vi "Classfy.vi"() -> (0 "Classfy 1":T1[](array[typedef])=[{"Item"="¤C¤H¨î¾ñÆV²y", "Count"=2, "Athletics"=["¨k¤l¤C¤H¨î¾ñÆV²y", "¤k¤l¤C¤H¨î¾ñÆV²y"]}, {"Item"="¤p½ü¨®", "Count"=2, "Athletics"=["¨k¤l­Ó¤H¤p½ü¨®", "¤k¤l­Ó¤H¤p½ü¨®"]}, {"Item"="¤½¸ô¦Û¥Ñ¨®", "Count"=4, "Athletics"=["¤k¤l­p®ÉÁÉ¤½¸ô¦Û¥Ñ¨®", "¨k¤l­p®ÉÁÉ¤½¸ô¦Û¥Ñ¨®", "¨k¤l¤½¸ôÁÉ¤½¸ô¦Û¥Ñ¨®", "¤k¤l¤½¸ôÁÉ¤½¸ô¦Û¥Ñ¨®"]}, {"Item"="¤â²y", "Count"=2, "Athletics"=["¨k¤l¤â²y", "¤k¤l¤â²y"]}, {"Item"="¤ô¤WªÝÁ¢", "Count"=2, "Athletics"=["¤k¤lÂù¤H¤ô¤WªÝÁ¢", "¤k¤l¹ÎÅé¤ô¤WªÝÁ¢"]}, {"Item"="¤ô²y", "Count"=2, "Athletics"=["¨k¤l¤ô²y", "¤k¤l¤ô²y"]}, {"Item"="¥Ð®|", "Count"=47, "Athletics"=["¨k¤l100¤½¤Ø", "¨k¤l200¤½¤Ø", "¨k¤l400¤½¤Ø", "¨k¤l800¤½¤Ø", "¨k¤l1500¤½¤Ø", "¨k¤l5000¤½¤Ø", "¨k¤l10,000¤½¤Ø", "¨k¤l110¤½¤Ø¸óÄæ", "¨k¤l400¤½¤Ø¸óÄæ", "¨k¤l3000¤½¤Ø»ÙÃª", "¨k¤l4¡Ñ100¤½¤Ø±µ¤O", "¨k¤l4¡Ñ400¤½¤Ø±µ¤O", "¨k¤l°¨©ÔªQ", "¨k¤l20¤½¨½Äv¨«", "¨k¤l50¤½¨½Äv¨«", "¨k¤l¸õ°ª", "¨k¤l¼µ¬ñ¸õ°ª", "¨k¤l¸õ»·", "¨k¤l¤T¯Å¸õ»·", "¨k¤l¹]²y", "¨k¤lÅK»æ", "¨k¤lÃì²y", "¨k¤l¼Ðºj", "¨k¤l¤Q¶µ¥þ¯à", "¤k¤l100¤½¤Ø", "¤k¤l200¤½¤Ø", "¤k¤l400¤½¤Ø", "¤k¤l800¤½¤Ø", "¤k¤l1500¤½¤Ø", "¤k¤l5000¤½¤Ø", "¤k¤l10,000¤½¤Ø", "¤k¤l100¤½¤Ø¸óÄæ", "¤k¤l400¤½¤Ø¸óÄæ", "¤k¤l3000¤½¤Ø»ÙÃª", "¤k¤l4¡Ñ100¤½¤Ø±µ¤O", "¤k¤l4¡Ñ400¤½¤Ø±µ¤O", "¤k¤l°¨©ÔªQ", "¤k¤l20¤½¨½Äv¨«", "¤k¤l¸õ°ª", "¤k¤l¼µ¬ñ¸õ°ª", "¤k¤l¸õ»·", "¤k¤l¤T¯Å¸õ»·", "¤k¤l¹]²y", "¤k¤lÅK»æ", "¤k¤lÃì²y", "¤k¤l¼Ðºj", "¤k¤l¤C¶µ¥þ¯à"]}, {"Item"="¦E²î", "Count"=14, "Athletics"=["¨k¤l³æ¤HÂù¼Õ", "¨k¤lÂù¤H³æ¼Õ", "¨k¤lÂù¤HÂù¼Õ", "¨k¤l¥|¤H³æ¼Õ", "¨k¤l¥|¤HÂù¼Õ", "¨k¤l¤K¤H³æ¼Õ", "¨k¤l»´¶q¯ÅÂù¤HÂù¼Õ", "¨k¤l»´¶q¯Å¥|¤H³æ¼Õ", "¤k¤l³æ¤HÂù¼Õ", "¤k¤lÂù¤H³æ¼Õ", "¤k¤lÂù¤HÂù¼Õ", "¤k¤l¥|¤HÂù¼Õ", "¤k¤l¤K¤H³æ¼Õ", "¤k¤l»´¶q¯ÅÂù¤HÂù¼Õ"]}, {"Item"="¦|²î", "Count"=10, "Athletics"=["¤k¤lRS¡GX«¬¡]­·®öªO¡^", "¤k¤l¹p®g¿ç®g«¬¡]³æ¤H¸¥¡^", "¤k¤l470«¬¡]Âù¤H¸¥¡^", "¤k¤l49¤H«¬FX¡]§Ö¸¥¡^", "¨k¤lRS¡GX«¬¡]­·®öªO¡^", "¨k¤l¹p®g«¬¡]³æ¤H¸¥¡^", "¨k¤lªâÄõ¤H«¬¡]³æ¤H¸¥¡^", "¨k¤l470«¬¡]Âù¤H¸¥¡^", "¨k¤l49¤H«¬¡]§Ö¸¥¡^", "²V¦XNacra17«¬¡]¦hÅé²î¡^"]}, {"Item"="¦±´Ò²y", "Count"=2, "Athletics"=["¨k¤l¦±´Ò²y", "¤k¤l¦±´Ò²y"]}, {"Item"="¦Ð²y", "Count"=5, "Athletics"=["²V¦XÂù¥´¦Ð²y", "¨k¤lÂù¥´¦Ð²y", "¤k¤lÂù¥´¦Ð²y", "¨k¤l³æ¥´¦Ð²y", "¤k¤l³æ¥´¦Ð²y"]}, {"Item"="¨FÅy±Æ²y", "Count"=2, "Athletics"=["¨k¤l¨FÅy±Æ²y", "¤k¤l¨FÅy±Æ²y"]}, {"Item"="¨¤¤O", "Count"=18, "Athletics"=["¨k¤l§ÆÃ¹¦¡59¤½¤ç¯Å", "¨k¤l§ÆÃ¹¦¡66¤½¤ç¯Å", "¨k¤l§ÆÃ¹¦¡75¤½¤ç¯Å", "¨k¤l§ÆÃ¹¦¡85¤½¤ç¯Å", "¨k¤l§ÆÃ¹¦¡98¤½¤ç¯Å", "¨k¤l§ÆÃ¹¦¡130¤½¤ç¯Å", "¨k¤l¦Û¥Ñ¦¡57¤½¤ç¯Å", "¨k¤l¦Û¥Ñ¦¡65¤½¤ç¯Å", "¨k¤l¦Û¥Ñ¦¡74¤½¤ç¯Å", "¨k¤l¦Û¥Ñ¦¡86¤½¤ç¯Å", "¨k¤l¦Û¥Ñ¦¡97¤½¤ç¯Å", "¨k¤l¦Û¥Ñ¦¡125¤½¤ç¯Å", "¤k¤l¦Û¥Ñ¦¡48¤½¤ç¯Å", "¤k¤l¦Û¥Ñ¦¡53¤½¤ç¯Å", "¤k¤l¦Û¥Ñ¦¡58¤½¤ç¯Å", "¤k¤l¦Û¥Ñ¦¡63¤½¤ç¯Å", "¤k¤l¦Û¥Ñ¦¡69¤½¤ç¯Å", "¤k¤l¦Û¥Ñ¦¡75¤½¤ç¯Å"]}, {"Item"="¨¬²y", "Count"=2, "Athletics"=["¨k¤l¨¬²y", "¤k¤l¨¬²y"]}, {"Item"="¬X¹D", "Count"=14, "Athletics"=["¨k¤l60¤½¤ç¯Å¬X¹D", "¨k¤l66¤½¤ç¯Å¬X¹D", "¨k¤l73¤½¤ç¯Å¬X¹D", "¨k¤l81¤½¤ç¯Å¬X¹D", "¨k¤l90¤½¤ç¯Å¬X¹D", "¨k¤l100¤½¤ç¯Å¬X¹D", "¨k¤l100¤½¤ç¥H¤W¯Å¬X¹D", "¤k¤l48¤½¤ç¯Å¬X¹D", "¤k¤l52¤½¤ç¯Å¬X¹D", "¤k¤l57¤½¤ç¯Å¬X¹D", "¤k¤l63¤½¤ç¯Å¬X¹D", "¤k¤l70¤½¤ç¯Å¬X¹D", "¤k¤l78¤½¤ç¯Å¬X¹D", "¤k¤l78¤½¤ç¥H¤W¯Å¬X¹D"]}, {"Item"="®g½b", "Count"=4, "Athletics"=["¨k¤l­Ó¤H®g½b", "¤k¤l­Ó¤H®g½b", "¨k¤l¹ÎÅé®g½b", "¤k¤l¹ÎÅé®g½b"]}, {"Item"="®gÀ»", "Count"=15, "Athletics"=["¨k¤l10¤½¤ØªÅ®ð¤âºj", "¨k¤l10¤½¤ØªÅ®ð¨Bºj", "¨k¤l25¤½¤Ø§Ö®g¤âºj", "¨k¤l50¤½¤Ø¤âºj", "¨k¤l50¤½¤Ø¨Bºjª×«º", "¨k¤l50¤½¤Ø¨Bºj¤T«º", "¨k¤l©w¦V­¸¹v", "¨k¤l¤£©w¦V­¸¹v", "¨k¤lÂù¤£©w¦V­¸¹v", "¤k¤l10¤½¤ØªÅ®ð¤âºj", "¤k¤l10¤½¤ØªÅ®ð¨Bºj", "¤k¤l25¤½¤Ø¤âºj", "¤k¤l50¤½¤Ø¨Bºj¤T«º", "¤k¤l©w¦V­¸¹v", "¤k¤l¤£©w¦V­¸¹v"]}, {"Item"="®±À»", "Count"=13, "Athletics"=["¨k¤l»´ÃÇ¶q49¤½¤ç¯Å", "¨k¤lÃÇ¶q52¤½¤ç¯Å", "¨k¤lÂú¶q56¤½¤ç¯Å", "¨k¤l»´¶q60¤½¤ç¯Å", "¨k¤l»´¨I¶q64¤½¤ç¯Å", "¨k¤l¨I¶q69¤½¤ç¯Å", "¨k¤l¤¤¶q75¤½¤ç¯Å", "¨k¤l»´­«¶q81¤½¤ç¯Å", "¨k¤l­«¶q91¤½¤ç¯Å", "¨k¤l¶W­«¶q91¤½¤ç¥H¤W¯Å", "¤k¤lÃÇ¶q51¤½¤ç¯Å", "¤k¤l»´¶q60¤½¤ç¯Å", "¤k¤l¤¤¶q75¤½¤ç¯Å"]}, {"Item"="®à²y", "Count"=4, "Athletics"=["¨k¤l³æ¥´®à²y", "¤k¤l³æ¥´®à²y", "¨k¤l¹ÎÅé®à²y", "¤k¤l¹ÎÅé®à²y"]}, {"Item"="°¨³N", "Count"=6, "Athletics"=["¹ÎÅé²±¸Ë»R¨BÁÉ", "­Ó¤H²±¸Ë»R¨BÁÉ", "­Ó¤H¤T¶µÁÉ", "¹ÎÅé¤T¶µÁÉ", "¹ÎÅé³õ¦a»ÙÃªÁÉ", "­Ó¤H³õ¦a»ÙÃªÁÉ"]}, {"Item"="蔼焊ひ", "Count"=2, "Athletics"=["¤k¤l­Ó¤H°ªº¸¤Ò", "¨k¤l­Ó¤H°ªº¸¤Ò"]}, {"Item"="±Æ²y", "Count"=2, "Athletics"=["¤k¤l±Æ²y", "¨k¤l±Æ²y"]}, {"Item"="²{¥N¤­¶µ", "Count"=2, "Athletics"=["¨k¤l­Ó¤H²{¥N¤­¶µ", "¤k¤l­Ó¤H²{¥N¤­¶µ"]}, {"Item"="³õ¦a¦Û¥Ñ¨®", "Count"=10, "Athletics"=["¨k¤l¹ÎÅéª§¥ýÁÉ", "¤k¤l¹ÎÅé°l³vÁÉ", "¨k¤l¹ÎÅé°l³vÁÉ", "¤k¤l¹ÎÅéª§¥ýÁÉ", "¨k¤lª§¥ýÁÉ", "¤k¤l°l³vÁÉ", "¨k¤l°l³vÁÉ", "¤k¤lª§¥ýÁÉ", "¨k¤l¥þ¯à", "¤k¤l¥þ¯à"]}, {"Item"="´åªa", "Count"=34, "Athletics"=["¨k¤l±¶ªa¡G50¤½¤Ø¡B100¤½¤Ø¡B200¤½¤Ø¡B400¤½¤Ø¡B1500¤½¤Ø", "¤k¤l±¶ªa¡G50¤½¤Ø¡B100¤½¤Ø¡B200¤½¤Ø¡B400¤½¤Ø¡B800¤½¤Ø", "¨k¤l¥õ¦¡¡G100¤½¤Ø¡B200¤½¤Ø", "¤k¤l¥õ¦¡¡G100¤½¤Ø¡B200¤½¤Ø", "¨k¤lµì¦¡¡G100¤½¤Ø¡B200¤½¤Ø", "¤k¤lµì¦¡¡G100¤½¤Ø¡B200¤½¤Ø", "¨k¤l½º¦¡¡G100¤½¤Ø¡B200¤½¤Ø", "¤k¤l½º¦¡¡G100¤½¤Ø¡B200¤½¤Ø", "¨k¤l²V¦X¦¡¡G200¤½¤Ø¡B400¤½¤Ø", "¤k¤l²V¦X¦¡¡G200¤½¤Ø¡B400¤½¤Ø", "¨k¤l±¶ªa±µ¤O¡G4¡Ñ100¤½¤Ø¡B4¡Ñ200¤½¤Ø", "¤k¤l±¶ªa±µ¤O¡G4¡Ñ100¤½¤Ø¡B4¡Ñ200¤½¤Ø", "¨k¤l²V¦X¦¡±µ¤O¡G4¡Ñ100¤½¤Ø", "¤k¤l²V¦X¦¡±µ¤O¡G4¡Ñ100¤½¤Ø", "¨k¤l¤½¶}¤ô°ì´åªa¡G10¤½¨½", "¤k¤l¤½¶}¤ô°ì´åªa¡G10¤½¨½"]}, {"Item"="µn¤s¦Û¥Ñ¨®", "Count"=2, "Athletics"=["¨k¤l¶V³¥ÁÉ", "¤k¤l¶V³¥ÁÉ"]}, {"Item"="¶`®±¹D", "Count"=8, "Athletics"=["¨k¤l58¤½¤ç¯Å¶`®±¹D", "¨k¤l68¤½¤ç¯Å¶`®±¹D", "¨k¤l80¤½¤ç¯Å¶`®±¹D", "¨k¤l80¤½¤ç¥H¤W¯Å¶`®±¹D", "¤k¤l49¤½¤ç¯Å¶`®±¹D", "¤k¤l57¤½¤ç¯Å ¶`®±¹D", "¤k¤l67¤½¤ç¯Å¶`®±¹D", "¤k¤l67¤½¤ç¥H¤W¯Å¶`®±¹D"]}, {"Item"="¸õ¤ô", "Count"=8, "Athletics"=["¤k¤l3¤½¤Ø¸õªO", "¤k¤l10¤½¤Ø¸õ¥x", "¤k¤lÂù¤H3¤½¤Ø¸õªO", "¤k¤lÂù¤H10¤½¤Ø¸õ¥x", "¨k¤l3¤½¤Ø¸õªO", "¨k¤l10¤½¤Ø¸õ¥x", "¨k¤lÂù¤H3¤½¤Ø¸õªO", "¨k¤lÂù¤H10¤½¤Ø¸õ¥x"]}, {"Item"="ºô²y", "Count"=5, "Athletics"=["¤k¤l³æ¥´ºô²y", "¤k¤lÂù¥´ºô²y", "¨k¤l³æ¥´ºô²y", "¨k¤lÂù¥´ºô²y", "²V¦XÂù¥´ºô²y"]}, {"Item"="»´¸¥¿E¬y", "Count"=4, "Athletics"=["¨k¤l³æ¤H¥[®³¤j¦¡¸¥", "¨k¤lÂù¤H¥[®³¤j¦¡¸¥", "¨k¤l³æ¤H·R´µ°ò¼¯¸¥", "¤k¤l³æ¤H·R´µ°ò¼¯¸¥"]}, {"Item"="»´¸¥Äv³t", "Count"=12, "Athletics"=["¨k¤l200¤½¤Ø³æ¤H¥[®³¤j¦¡¸¥", "¨k¤l1000¤½¤Ø³æ¤H¥[®³¤j¦¡¸¥", "¨k¤l1000¤½¤ØÂù¤H¥[®³¤j¦¡¸¥", "¨k¤l200¤½¤Ø³æ¤H·R´µ°ò¼¯¸¥", "¨k¤l1000¤½¤Ø³æ¤H·R´µ°ò¼¯¸¥", "¨k¤l200¤½¤ØÂù¤H·R´µ°ò¼¯¸¥", "¨k¤l1000¤½¤ØÂù¤H·R´µ°ò¼¯¸¥", "¨k¤l1000¤½¤Ø¥|¤H·R´µ°ò¼¯¸¥", "¤k¤l500¤½¤Ø³æ¤H·R´µ°ò¼¯¸¥", "¤k¤l500¤½¤ØÂù¤H·R´µ°ò¼¯¸¥", "¤k¤l500¤½¤Ø¥|¤H·R´µ°ò¼¯¸¥", "¤k¤l200¤½¤Ø³æ¤H·R´µ°ò¼¯¸¥"]}, {"Item"="¼uÂ½§É", "Count"=2, "Athletics"=["¨k¤l­Ó¤H¼uÂ½§É", "¤k¤l­Ó¤H¼uÂ½§É"]}, {"Item"="À»¼C", "Count"=10, "Athletics"=["¤k¤l¶w¼C­Ó¤HÁÉ", "¨k¤l¶w¼C­Ó¤HÁÉ", "¨k¤l¶w¼C¹ÎÅéÁÉ", "¤k¤l¾U¼C­Ó¤HÁÉ", "¨k¤l¾U¼C­Ó¤HÁÉ", "¤k¤l¾U¼C¹ÎÅéÁÉ", "¤k¤l­x¤M­Ó¤HÁÉ", "¨k¤l­x¤M­Ó¤HÁÉ", "¤k¤l­x¤M¹ÎÅéÁÉ", "¨k¤l­x¤M¹ÎÅéÁÉ"]}, {"Item"="Á|­«", "Count"=15, "Athletics"=["¨k¤l56¤½¤ç¯ÅÁ|­«", "¨k¤l62¤½¤ç¯ÅÁ|­«", "¨k¤l69¤½¤ç¯ÅÁ|­«", "¨k¤l77¤½¤ç¯ÅÁ|­«", "¨k¤l85¤½¤ç¯ÅÁ|­«", "¨k¤l94¤½¤ç¯ÅÁ|­«", "¨k¤l105¤½¤ç¯ÅÁ|­«", "¨k¤l105¤½¤ç¥H¤W¯ÅÁ|­«", "¤k¤l48¤½¤ç¯ÅÁ|­«", "¤k¤l53¤½¤ç¯ÅÁ|­«", "¤k¤l58¤½¤ç¯ÅÁ|­«", "¤k¤l63¤½¤ç¯ÅÁ|­«", "¤k¤l69¤½¤ç¯ÅÁ|­«", "¤k¤l75¤½¤ç¯ÅÁ|­«", "¤k¤l75¤½¤ç¥H¤W¯ÅÁ|­«"]}, {"Item"="Ãý«ßÅé¾Þ", "Count"=2, "Athletics"=["¤k¤l­Ó¤H¥þ¯àÃý«ßÅé¾Þ", "¤k¤l¹ÎÅé¥þ¯àÃý«ßÅé¾Þ"]}, {"Item"="Äv§ÞÅé¾Þ", "Count"=14, "Athletics"=["¨k¤l­Ó¤H¥þ¯àÄv§ÞÅé¾Þ", "¨k¤l¹ÎÅéÄv§ÞÅé¾Þ", "¨k¤l¸õ°¨", "¨k¤l¦Û¥ÑÅé¾Þ", "¨k¤l¾b°¨", "¨k¤l¦QÀô", "¨k¤lÂùºb", "¨k¤l³æºb", "¤k¤l­Ó¤H¥þ¯àÄv§ÞÅé¾Þ", "¤k¤l¹ÎÅéÄv§ÞÅé¾Þ", "¤k¤l¸õ°¨", "¤k¤l¥­¿Å¤ì", "¤k¤l°ª§Cºb", "¤k¤l¦Û¥ÑÅé¾Þ"]}, {"Item"="Äx²y", "Count"=2, "Athletics"=["¨k¤lÄx²y", "¤k¤lÄx²y"]}, {"Item"="ÅK¤H¤T¶µ", "Count"=2, "Athletics"=["¨k¤l­Ó¤HÅK¤H¤T¶µ", "¤k¤l­Ó¤HÅK¤H¤T¶µ"]}, {"Item"="Á`¼Æ", "Count"=306, "Athletics"=[]}])   [LabVIEW 2015]
uses:
  Data Def/Classify.ctl
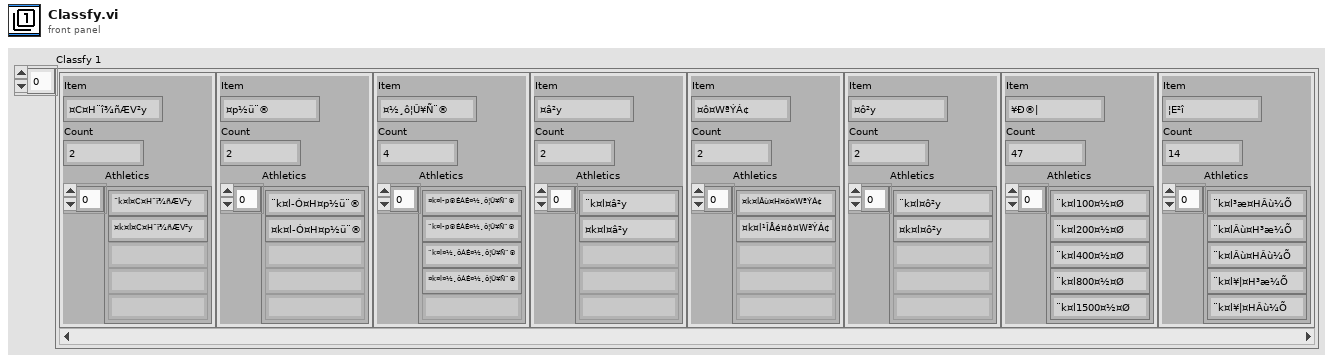
[diagram p1: front panel]
types:
  T1 = typedef "Classify.ctl" = cluster{"Item":string, "Count":i32, "Athletics":string[]}
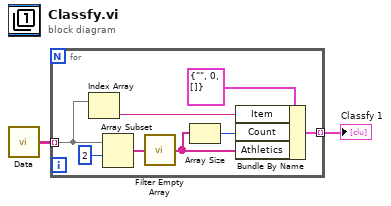
[diagram p0: block diagram]
diagram:
  n1 = call "Data.vi"() -> ("Data"=w1:string[][])
  n2 = for {
    tunnel: [w8] -> w2 mode=indexing
    tunnel: w1 -> [w5] mode=indexing
    n3 = Index Array(array=w5) -> (element=w4:string)  [unwired: 1 in]
    n4 = Array Subset(array=w5, index=2) -> (w3:string[])  [unwired: 1 in]
    n5 = call "Filter Empty Array.vi"("Array In"=w3) -> ("Array Out"=w7:string[])
    n6 = Array Size(array=w7) -> (size(s)=w6:i32)
    n7 = Bundle By Name(cluster=T1 {"Item"="", "Count"=0, "Athletics"=[]} ("Classify 1"), "Item"=w4, "Count"=w6, "Athletics"=w7) -> (w8:T1)
  }
  "Classfy 1" <- w2
